vi "Close Connection.vi"(8 "error in (no error)":errorcluster, 11 "sqlite in":refnum<class "sqlite3.lvclass">) -> (0 "error out":errorcluster, 3 "sqlite out":refnum<class "sqlite3.lvclass">)   [LabVIEW 2020, in "sqlite3.lvlib" / "sqlite3.lvclass"]
uses:
  sqlite3.lvclass
  sqlite3.lvclass/sqlite3.ctl
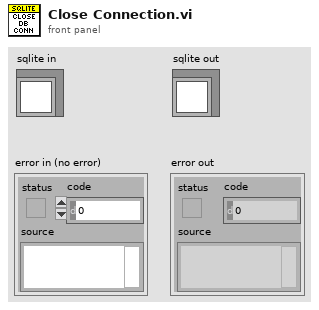
[diagram p1: front panel]
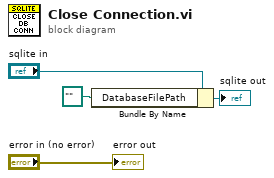
[diagram p0: block diagram]
diagram:
  n1 = Bundle By Name(cluster="sqlite in", "DatabaseFilePath"=path "") -> (→"sqlite out":refnum<class "sqlite3.lvclass">)
  "error out" <- "error in (no error)"
